vi "Write stop.vi"(8 "error in (no error)":errorcluster, 10 "stop":refnum<user-event>, 11 "Monochromator in":refnum<class "Monochromator.lvclass">) -> (0 "error out":errorcluster, 3 "Monochromator out":refnum<class "Monochromator.lvclass">)   [LabVIEW 2016, in "Monochromator.lvclass"]
uses:
  Monochromator.lvclass
  Monochromator.lvclass/Monochromator.ctl
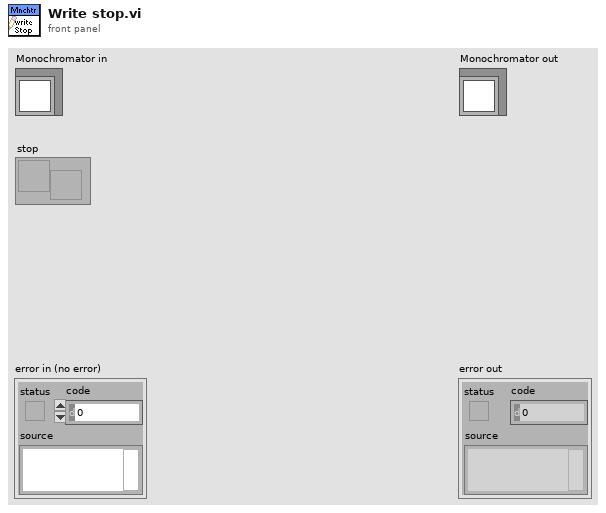
[diagram p1: front panel]
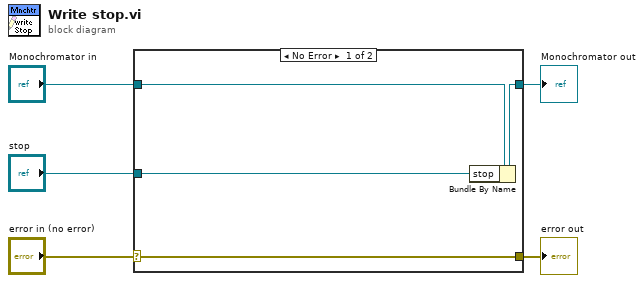
[diagram p0: block diagram]
diagram:
  n1 = case shown="No Error" "error in (no error)" {
    selector: "error in (no error)" -> [w9 w10]
    tunnel: [w9 w10] -> w4
    tunnel: [w7 w11] -> w2
    tunnel: "Monochromator in" -> [w8 w11]
    tunnel: "stop" -> [w6 _]
    frame No Error {
      n2 = Bundle By Name(cluster=w8, "stop"=w6) -> (w7:refnum<class "Monochromator.lvclass">)
    }
    frame Error {
    }
  }
  "error out" <- w4
  "Monochromator out" <- w2
